vi "parseBMSPDO.vi"(8 "error in (no error)":errorcluster, 9 "PDO channel":u8(ring) items=["PDO 1", "PDO 2", "PDO 3", "PDO 4"], 10 "TPDO data":u8[](array[numeric]) format="%x", 11 "OrionBMS in":refnum<class "OrionBMSClass.lvclass">) -> (0 "error out":errorcluster, 3 "OrionBMS out":refnum<class "OrionBMSClass.lvclass">)   [LabVIEW 2018, in "OrionBMSClass.lvclass"]
uses:
  OrionBMSClass.lvclass
  <vilib>/CANopenLib/CANOPEN.llb/CANopen Fetch from Data [U16].vi
  <vilib>/CANopenLib/CANOPEN.llb/CANopen Fetch from Data [I8].vi
  <vilib>/CANopenLib/CANOPEN.llb/CANopen Fetch from Data [I16].vi
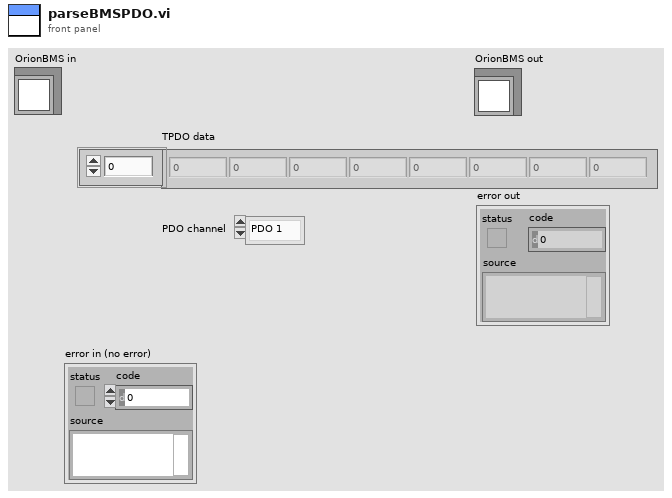
[diagram p1: front panel]
types:
  T1 = typedef "TypeDef_BMSDatas.ctl" = cluster{"Pack 1 Max Cell\n Voltage (V)":dbl, "Pack 1 Max Cell\n ID ":dbl, "Pack 1 Min Cell \nVoltage (V)":dbl, "Pack 1 Min Cell \nID ":dbl, "Pack 1 State of Charge  (%)":dbl, "Pack 1 Average Voltage1 (V)":dbl, "Pack 1Voltage Delta (V)":dbl, "Pack 1 Current (A)":dbl, "Pack 1 Voltage (V)":dbl, "Pack 1 Max Resistance (Ohm)":dbl, "Pack 1Min Resistance (Ohm)":dbl, "Pack 1Average Resistance (Ohm)":dbl, "Pack 1Delta Resistance (Ohm)":dbl, "Pack 1 Highest Temperature(F)":dbl, "BmsStatus1":T2, "Pack 2 Max Cell\n Voltage (V) ":dbl, "Pack 2 Max Cell\n ID  ":dbl, "Pack 2 Min Cell \nVoltage (V) ":dbl, "Pack 2 Min Cell \nID  ":dbl, "Pack 2 Average Voltage1 (V)":dbl, "Pack 2 Voltage Delta (V) ":dbl, "Pack 2 Current (A)":dbl, "Pack 2 Voltage (V) ":dbl, "Pack 2 State of Charge  (%) ":dbl, "Pack 2 Max Resistance (Ohm) ":dbl, "Pack 2 Min Resistance (Ohm)":dbl, "Pack 2 Average Resistance (Ohm)":dbl, "Pack 2 Delta Resistance (Ohm) ":dbl, "Pack 2 Highest Temperature(F) ":dbl, "BmsStatus 2":T2}
  T2 = typedef "TypeDef_BMSStatuss.ctl" = cluster{"isFault":bool, "isolationMonitoring":bool}
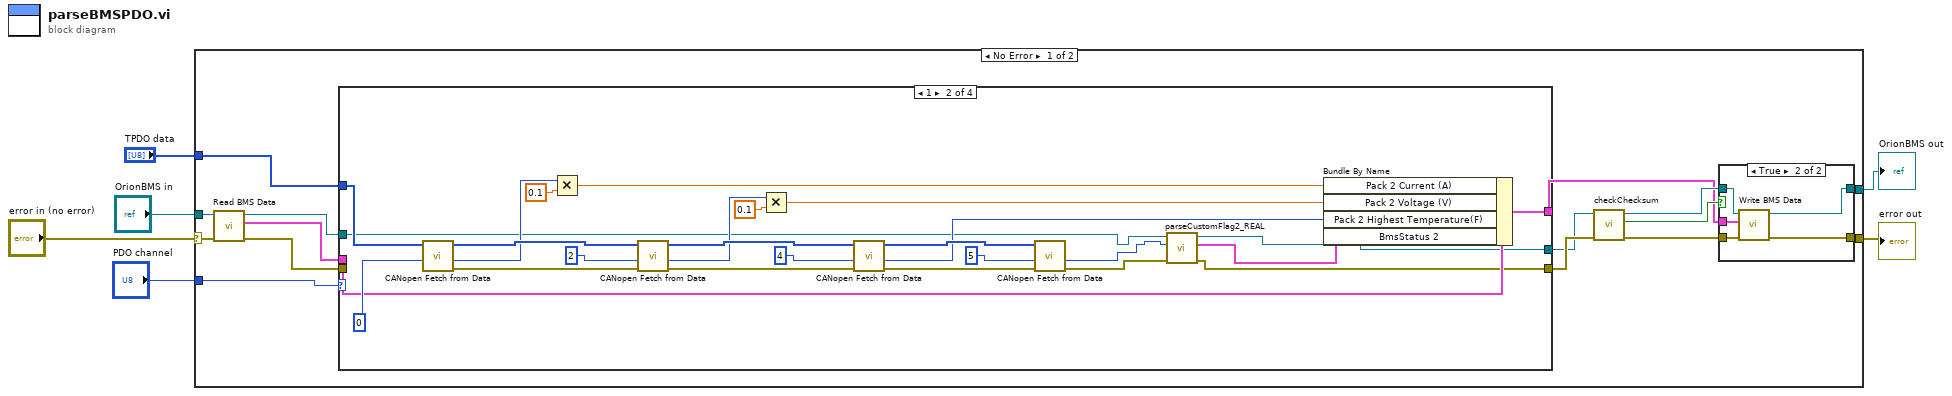
[diagram p0: block diagram]
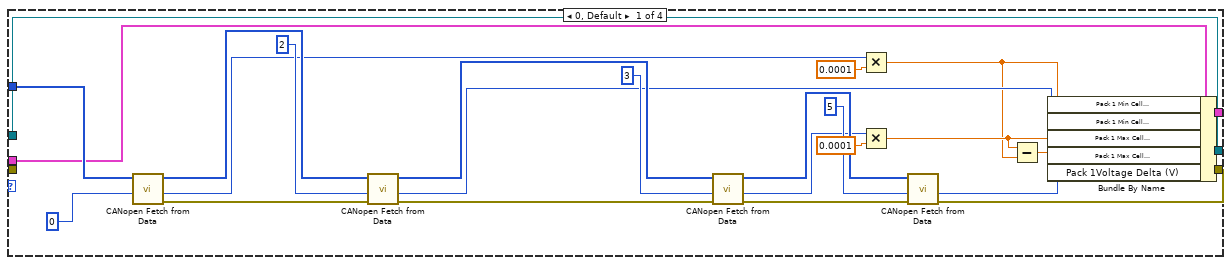
[diagram p3: hidden frame]
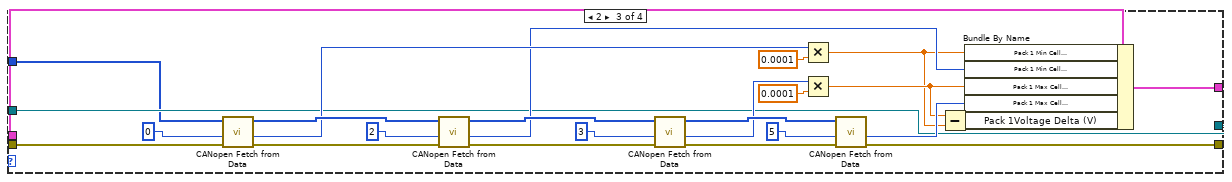
[diagram p4: hidden frame]
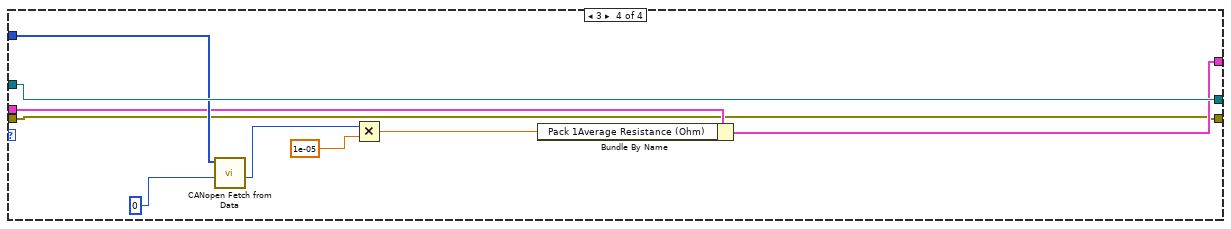
[diagram p5: hidden frame]
diagram:
  n1 = case shown="No Error" "error in (no error)" {
    selector: "error in (no error)" -> [w20 w113]
    tunnel: "OrionBMS in" -> [w21 w114]
    tunnel: "TPDO data" -> [w7 _]
    tunnel: "PDO channel" -> [w19 _]
    tunnel: [w14 w114] -> w2
    tunnel: [w13 w113] -> w1
    frame No Error {
      n2 = call-dynamic "Read BMS Data.vi"("error in (no error)"=w20, "OrionBMS in"=w21) -> ("error out"=w11:errorcluster, "BMS Data"=w18:T1, "OrionBMS out"=w9:refnum<class "OrionBMSClass.lvclass">)  [unwired: 7 in]
      n3 = case shown="1" w19 {
        tunnel: w18 -> [w31 w64 w82 w108]
        tunnel: [w29 w55 w83 w105] -> w17
        tunnel: w11 -> [_ _ w84 w105]
        tunnel: [w30 w60 w81 w106] -> w8
        tunnel: [w52 w53 w80 w112] -> w10
        tunnel: w9 -> [w52 w58 w80 w112]
        tunnel: w7 -> [w32 w59 w79 w110]
        frame 0, Default {
          n4 = call-poly <vilib>:"CANopen Fetch from Data.vi"("offset (0)"=u32 0, "CANopen data in"=w32) -> ("error out"=w47:errorcluster, "unsigned 16-bit integer"=w40:u16, "CANopen data out"=w51:u8[])  [unwired: 7 in]
          n5 = call-poly <vilib>:"CANopen Fetch from Data.vi"("error in (no error)"=w47, "offset (0)"=u32 2, "CANopen data in"=w51) -> ("error out"=w46:errorcluster, "signed 8-bit integer"=w39:i8, "CANopen data out"=w42:u8[])  [unwired: 6 in]
          n6 = call-poly <vilib>:"CANopen Fetch from Data.vi"("error in (no error)"=w46, "offset (0)"=u32 3, "CANopen data in"=w42) -> ("error out"=w45:errorcluster, "unsigned 16-bit integer"=w38:u16, "CANopen data out"=w43:u8[])  [unwired: 6 in]
          n7 = Multiply(x=w40, y=0.0001) -> (x*y=w34:dbl)
          n8 = Multiply(x=w38, y=0.0001) -> (x*y=w35:dbl)
          n9 = call-poly <vilib>:"CANopen Fetch from Data.vi"("error in (no error)"=w45, "offset (0)"=u32 5, "CANopen data in"=w43) -> ("error out"=w29:errorcluster, "signed 8-bit integer"=w36:i8)  [unwired: 6 in, 1 out]
          n10 = Subtract(x=w35, y=w34) -> (x-y=w33:dbl)
          n11 = Bundle By Name(cluster=w31, "Pack 1 Min Cell \nVoltage (V)"=w34, "Pack 1 Min Cell \nID"=w39, "Pack 1 Max Cell\n Voltage (V)"=w35, "Pack 1 Max Cell\n ID"=w36, "Pack 1Voltage Delta (V)"=w33) -> (w30:T1)
        }
        frame 1 {
          n12 = call-poly <vilib>:"CANopen Fetch from Data.vi"("offset (0)"=u32 0, "CANopen data in"=w59) -> ("error out"=w74:errorcluster, "unsigned 16-bit integer"=w67:u16, "CANopen data out"=w78:u8[])  [unwired: 7 in]
          n13 = Multiply(x=w67, y=0.1) -> (x*y=w63:dbl)
          n14 = call-poly <vilib>:"CANopen Fetch from Data.vi"("error in (no error)"=w74, "offset (0)"=u32 2, "CANopen data in"=w78) -> ("error out"=w73:errorcluster, "signed 16-bit integer"=w65:i16, "CANopen data out"=w69:u8[])  [unwired: 6 in]
          n15 = Multiply(x=w65, y=0.1) -> (x*y=w62:dbl)
          n16 = call-poly <vilib>:"CANopen Fetch from Data.vi"("error in (no error)"=w73, "offset (0)"=u32 4, "CANopen data in"=w69) -> ("error out"=w72:errorcluster, "signed 8-bit integer"=w61:i8, "CANopen data out"=w70:u8[])  [unwired: 6 in]
          n17 = call-poly <vilib>:"CANopen Fetch from Data.vi"("error in (no error)"=w72, "offset (0)"=u32 5, "CANopen data in"=w70) -> ("error out"=w56:errorcluster, "signed 8-bit integer"=w57:i8)  [unwired: 6 in, 1 out]
          n18 = call "parseCustomFlag2_REAL.vi"("error in (no error)"=w56, "Numeric"=w57, "OrionBMS in"=w58) -> ("error out"=w55:errorcluster, "output cluster"=w54:T2, "OrionBMS out"=w53:refnum<class "OrionBMSClass.lvclass">)  [unwired: 6 in]
          n19 = Bundle By Name(cluster=w64, "Pack 2 Current (A)"=w63, "Pack 2 Voltage (V)"=w62, "Pack 2 Highest Temperature(F)"=w61, "BmsStatus 2"=w54) -> (w60:T1)
        }
        frame 2 {
          n20 = call-poly <vilib>:"CANopen Fetch from Data.vi"("error in (no error)"=w84, "offset (0)"=u32 0, "CANopen data in"=w79) -> ("error out"=w99:errorcluster, "unsigned 16-bit integer"=w92:u16, "CANopen data out"=w103:u8[])  [unwired: 6 in]
          n21 = call-poly <vilib>:"CANopen Fetch from Data.vi"("error in (no error)"=w99, "offset (0)"=u32 2, "CANopen data in"=w103) -> ("error out"=w98:errorcluster, "signed 8-bit integer"=w91:i8, "CANopen data out"=w94:u8[])  [unwired: 6 in]
          n22 = call-poly <vilib>:"CANopen Fetch from Data.vi"("error in (no error)"=w98, "offset (0)"=u32 3, "CANopen data in"=w94) -> ("error out"=w97:errorcluster, "unsigned 16-bit integer"=w90:u16, "CANopen data out"=w95:u8[])  [unwired: 6 in]
          n23 = Multiply(x=w92, y=0.0001) -> (x*y=w86:dbl)
          n24 = Multiply(x=w90, y=0.0001) -> (x*y=w87:dbl)
          n25 = call-poly <vilib>:"CANopen Fetch from Data.vi"("error in (no error)"=w97, "offset (0)"=u32 5, "CANopen data in"=w95) -> ("error out"=w83:errorcluster, "signed 8-bit integer"=w88:i8)  [unwired: 6 in, 1 out]
          n26 = Subtract(x=w87, y=w86) -> (x-y=w85:dbl)
          n27 = Bundle By Name(cluster=w82, "Pack 1 Min Cell \nVoltage (V)"=w86, "Pack 1 Min Cell \nID"=w91, "Pack 1 Max Cell\n Voltage (V)"=w87, "Pack 1 Max Cell\n ID"=w88, "Pack 1Voltage Delta (V)"=w85) -> (w81:T1)
        }
        frame 3 {
          n28 = call-poly <vilib>:"CANopen Fetch from Data.vi"("offset (0)"=u32 0, "CANopen data in"=w110) -> ("signed 16-bit integer"=w104:i16)  [unwired: 7 in, 2 out]
          n29 = Multiply(x=w104, y=1e-05) -> (x*y=w107:dbl)
          n30 = Bundle By Name(cluster=w108, "Pack 1Average Resistance (Ohm)"=w107) -> (w106:T1)
        }
      }
      n31 = call "checkChecksum.vi"("error in (no error)"=w17, "OrionBMS in"=w10) -> ("error in (no error) 2"=w16:errorcluster, "checkSumMatched"=w12:bool, "OrionBMS out"=w15:refnum<class "OrionBMSClass.lvclass">)  [unwired: 7 in]
      n32 = case shown="True" w12 {
        tunnel: w16 -> [w22 w28]
        tunnel: w15 -> [w23 w27]
        tunnel: [w23 w26] -> w14
        tunnel: [w22 w25] -> w13
        tunnel: w8 -> [_ w24]
        frame False {
        }
        frame True {
          n33 = call-dynamic "Write BMS Data.vi"("error in (no error)"=w28, "BMS Data"=w24, "OrionBMS in"=w27) -> ("error out"=w25:errorcluster, "OrionBMS out"=w26:refnum<class "OrionBMSClass.lvclass">)  [unwired: 7 in]
        }
      }
    }
    frame Error {
    }
  }
  "OrionBMS out" <- w2
  "error out" <- w1
